vi "UpdateTag.vi"(8 "error in (no error)":errorcluster, 10 "CreateNameTag":string, 11 "ClassDataTree in":refnum<class "ClassDataTree.lvclass">) -> (0 "error out":errorcluster, 3 "ClassDataTree out":refnum<class "ClassDataTree.lvclass">)   [LabVIEW 2016, in "ClassDataTree.lvclass"]
uses:
  ClassDataTree.lvclass
  ClassDataTree.lvclass/ClassDataTree.ctl
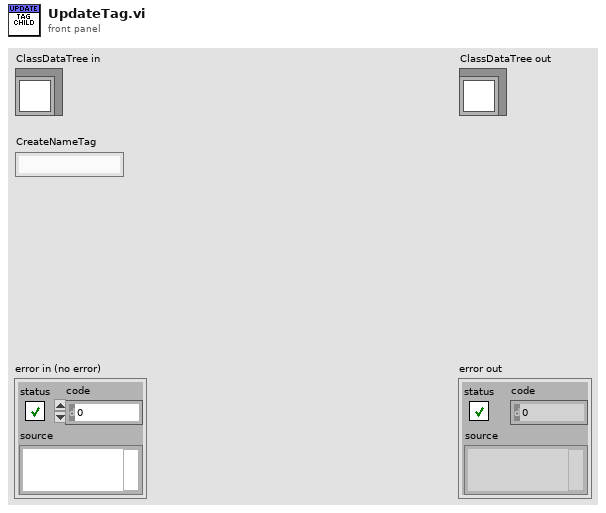
[diagram p1: front panel]
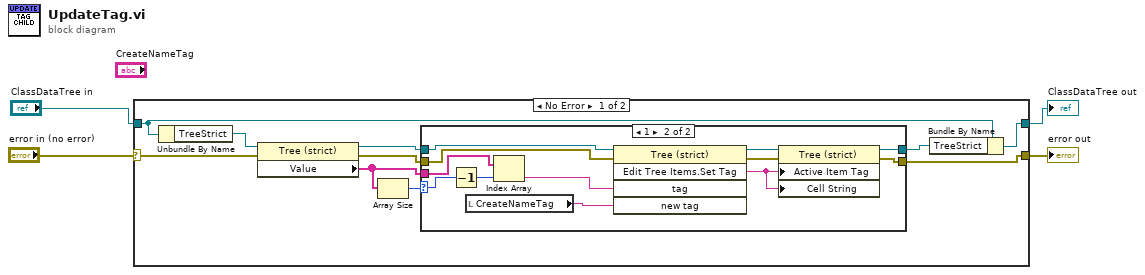
[diagram p0: block diagram]
diagram:
  n1 = case shown="No Error" "error in (no error)" {
    selector: "error in (no error)" -> [w13 w30]
    tunnel: [w6 w30] -> w3
    tunnel: [w11 w29] -> w1
    tunnel: "ClassDataTree in" -> [w12 w29]
    frame No Error {
      n2 = Unbundle By Name(w12) -> ("TreeStrict"=w14:refnum<vi>)
      n3 = property class="Tree (strict)"(reference=w14, error in=w13) -> (reference out=w9:refnum<vi>, error out=w8:errorcluster, "Value"=w5:string[])
      n4 = Array Size(array=w5) -> (size(s)=w10:i32)
      n5 = case shown="1" w10 {
        selector: w10 -> [_ w22]
        tunnel: w9 -> [w16 w28]
        tunnel: w8 -> [w15 w27]
        tunnel: [w16 w18] -> w7
        tunnel: [w15 w17] -> w6
        tunnel: w5 -> [_ w26]
        frame 0, Default {
        }
        frame 1 {
          n6 = Decrement(x=w22) -> (x-1=w23:i32)
          n7 = local read "CreateNameTag"() -> (w24:string)
          n8 = Index Array(array=w26, index=w23) -> (element=w25:string)
          n9 = invoke class="Tree (strict)" method="Edit Tree Items.Set Tag"(reference=w28, error in=w27, "tag"=w25, "new tag"=w24) -> (reference out=w21:refnum<vi>, error out=w19:errorcluster, "Edit Tree Items:Set Tag"=w20:string)  [unwired: 1 in, 2 out]
          n10 = property class="Tree (strict)"(reference=w21, error in=w19, "Active Item Tag"=w20, "Cell String"=w20) -> (reference out=w18:refnum<vi>, error out=w17:errorcluster)
        }
      }
      n11 = Bundle By Name(cluster=w12, "TreeStrict"=w7) -> (w11:refnum<class "ClassDataTree.lvclass">)
    }
    frame Error {
    }
  }
  "error out" <- w3
  "ClassDataTree out" <- w1
